vi "main2work.vi"() -> ()   [LabVIEW 2014]
uses:
  type definitions/control camera properties.ctl
  type definitions/state machine enum.ctl
  <vilib>/userdefined/High Color/IMAQdx.ctl
  <vilib>/vision/driver/NI_Vision_Acquisition_Software.lvlib
panel:
  in  "Control Camera Properties":T1={"Packet Size"=1500, "Pixel Format"=17825797, "Gain in dB"=1.0, "Exposure Time in µs"=1500, "Stream MBytes per Second"=124} {"Stream MBytes per Second" min=1 max=124 step=1 format="%#.6p"; "Exposure Time in µs" min=21 max=153391689 format="%#.0f"; "Gain in dB" min=0.0 max=26.0 format="%#_2g"; "Pixel Format" items=["Mono 12 Packed"=17563654, "Mono 12"=17825797, "Mono 8"=17301505]}
  in  "Stop Grab 2":bool
  out "Image":T2(plugin-control)
  in  "Calibration Button":bool
  out "Image Pixels (I16)":i16[][](array[numeric])
  out "Camera":T3
  in  "select camera":bool
  in  "Stop Button":bool
  in  "Snap Button":bool
  in  "Grab Button":bool
  in  "Save As Button":bool
  in  "Save Button":bool
  # "Bytes"
  # "Trigger"
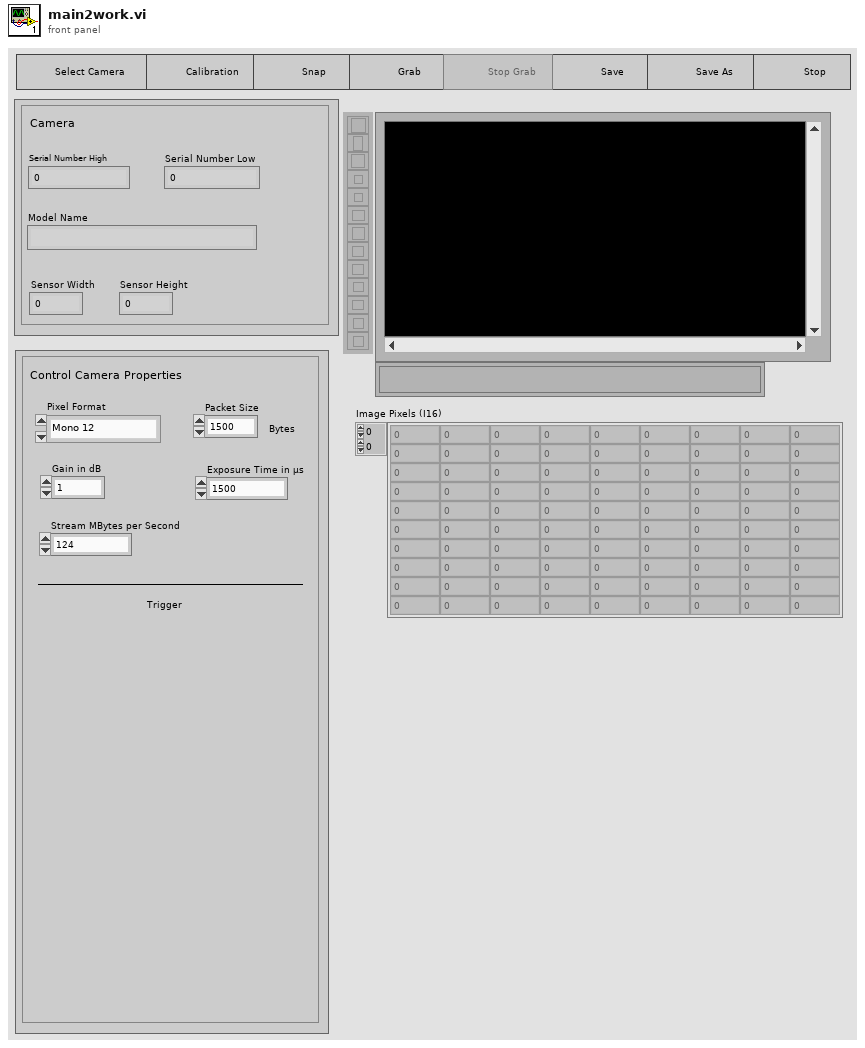
[diagram p1: front panel]
types:
  T1 = typedef "control camera properties.ctl" = cluster{"Packet Size":u32, "Pixel Format":u32, "Gain in dB":dbl, "Exposure Time in µs":u32, "Stream MBytes per Second":u32}
  T2 = typedef "IMAQ Image.ctl" = refnum<image>
  T3 = cluster{"Serial Number High":u32, "Model Name":string, "Sensor Width":u32, "Sensor Height":u32, "Serial Number Low":u32}
  T4 = cluster{"Packet Size":u32, "Pixel Format":u32, "Gain in dB":dbl, "Exposure Time in µs":u32, "Stream Bytes per Second":u32}
  T5 = typedef "IMAQdx.ctl" = refnum<k21>
  T6 = typedef "state machine enum.ctl" = enum16{"start", "select camera", "control camera properties", "calibration", "wait", "snap", "save", "save as", "grab", "error", "stop"}
  T7 = enum8{"Enabled", "Disabled", "Disabled and Grayed Out"}
  T8 = cluster{"Serial Number High":bool, "Model Name":bool, "Sensor Width":bool, "Sensor Height":bool, "Serial Number Low":bool}
  T9 = typedef "Image Type" = u32
  T10 = cluster{"PixelFormat":u32, "PacketSize":u32, "ValueDBL":dbl, "ValueU32":u32, "ValueU32":u32}
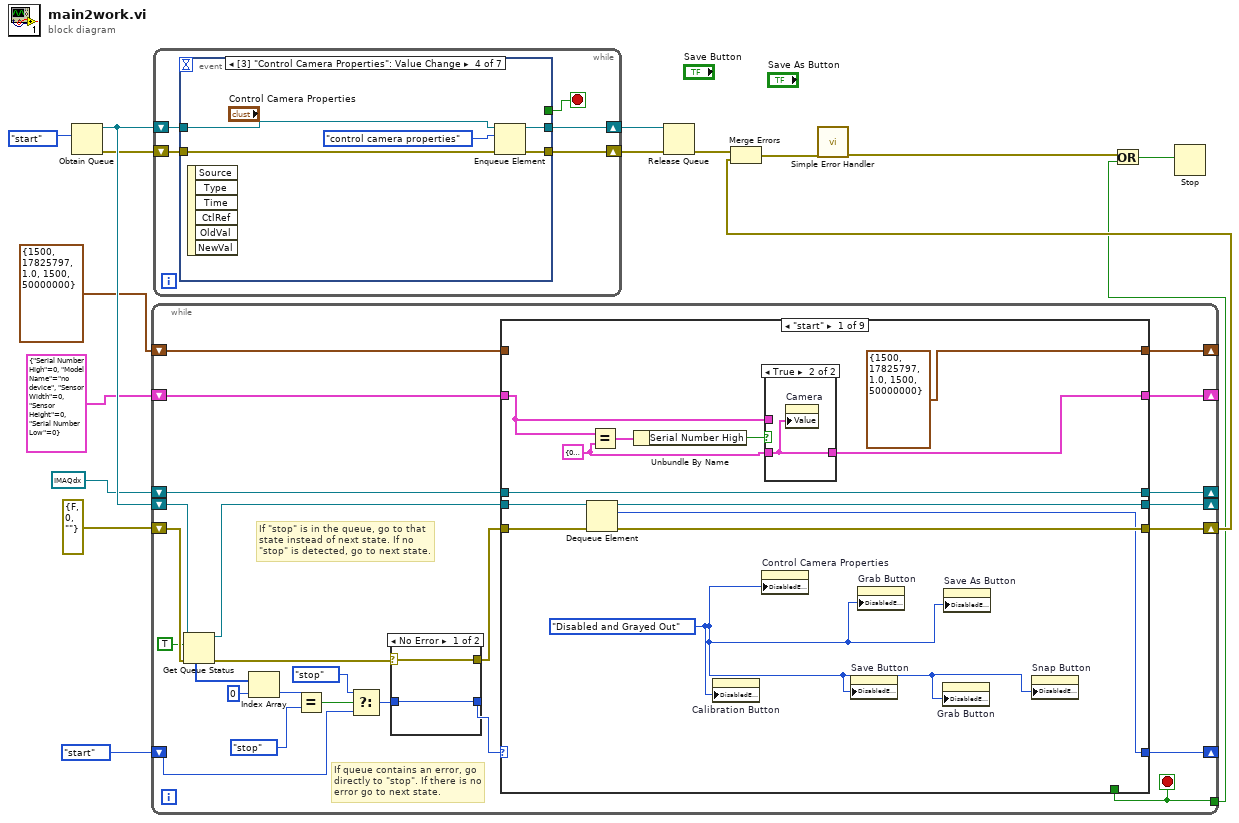
[diagram p0: block diagram]
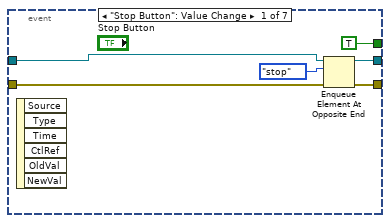
[diagram p2: hidden frame]
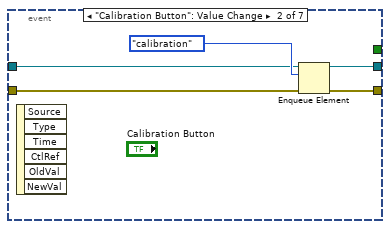
[diagram p3: hidden frame]
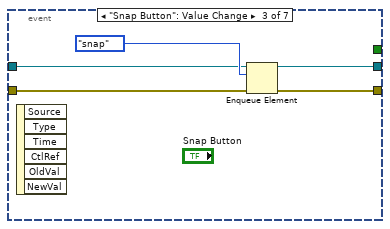
[diagram p4: hidden frame]
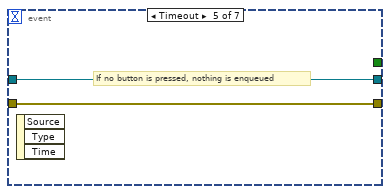
[diagram p5: hidden frame]
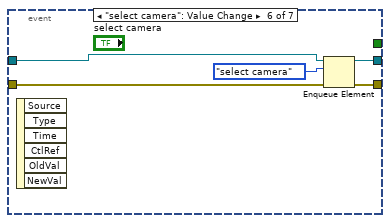
[diagram p6: hidden frame]
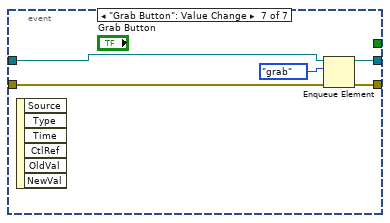
[diagram p7: hidden frame]
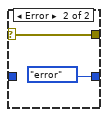
[diagram p8: hidden frame]
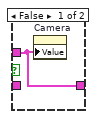
[diagram p9: hidden frame]
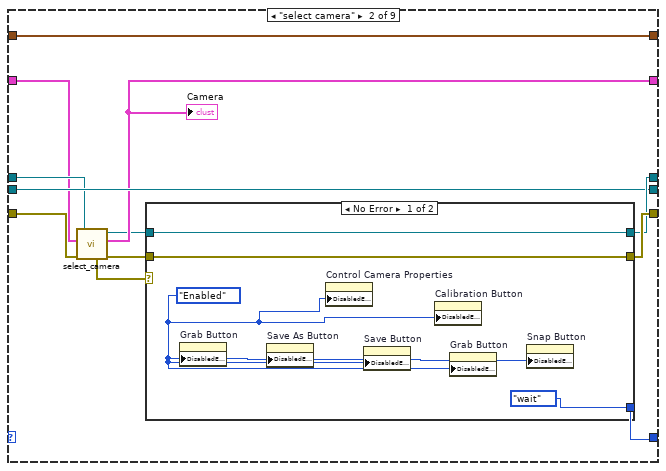
[diagram p10: hidden frame]
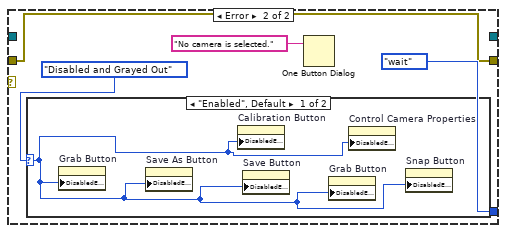
[diagram p11: hidden frame]
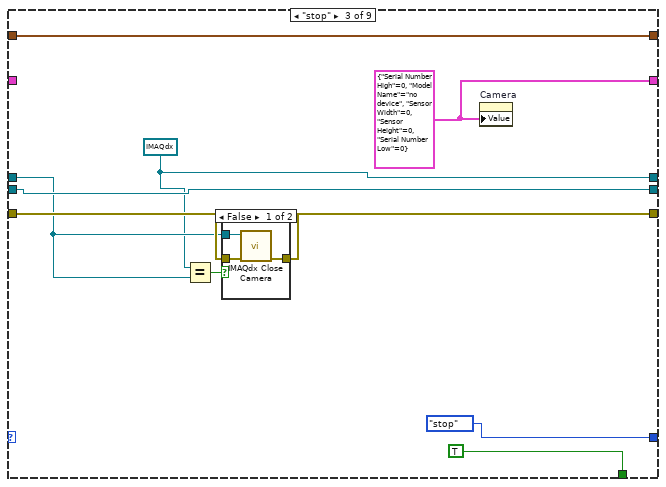
[diagram p13: hidden frame]
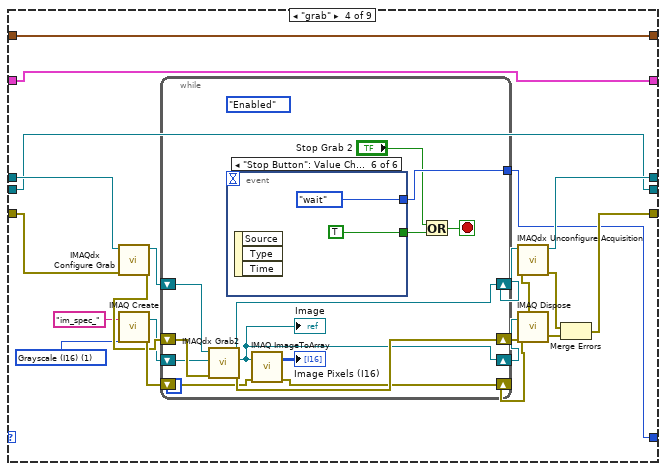
[diagram p15: hidden frame]
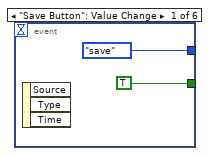
[diagram p16: hidden frame]
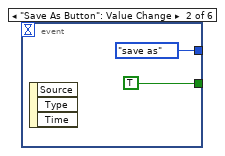
[diagram p17: hidden frame]
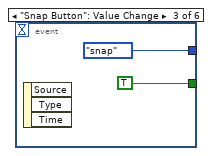
[diagram p18: hidden frame]
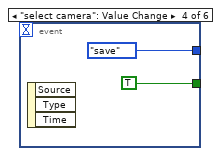
[diagram p19: hidden frame]
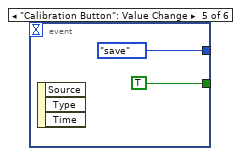
[diagram p20: hidden frame]
diagram:
  n1 = Obtain Queue(element data type=state_machine_enum."start" ("Zustände")) -> (queue out=w15:refnum<queue>, error out=w5:errorcluster)  [unwired: 4 in, 1 out]
  n2 = while {
    shift-right: [w17] -> _
    shift-left: T4 {"Packet Size"=1500, "Pixel Format"=17825797, "Gain in dB"=1.0, "Exposure Time in µs"=1500, "Stream Bytes per Second"=50000000} ("Control Camera Properties 3") -> [w41]
    shift-right: [w37] -> w11
    shift-left: errorcluster {"status"=FALSE, "code"=0, "source"=""} ("error out") -> [w32]
    shift-right: [w40] -> _
    shift-left: state_machine_enum."start" ("Zustände") -> [w25]
    shift-right: [w39] -> _
    shift-left: T5 refnum ("Session Out 2") -> [w38]
    shift-right: [w36] -> _
    shift-left: w15 -> [w34]
    tunnel: [w35] -> w4
    shift-right: [w19] -> _
    shift-left: T3 {"Serial Number High"=0, "Model Name"="no device", "Sensor Width"=0, "Sensor Height"=0, "Serial Number Low"=0} ("Camera 2") -> [w18]
    stop <- w35 stop-if-true
    # "If queue contains an error, go\ndirectly to \"stop\". If there is no\nerror go to next state."
    # "If \"stop\" is in the queue, go to that \nstate instead of next state. If no\n\"stop\" is detected, go to next state."
    n3 = Get Queue Status(queue=w34, return elements? (F)=TRUE, error in (no error)=w32) -> (queue out=w33:refnum<queue>, error out=w23:errorcluster, elements=w28:T6[])  [unwired: 5 out]
    n4 = Index Array(array=w28, index=0) -> (element=w30:T6)
    n5 = Equal?(x=w30, y=state_machine_enum."stop" ("Zustände")) -> (x = y?=w31:bool)
    n6 = Select(t=state_machine_enum."stop" ("Zustände"), s=w31, f=w25) -> (s? t:f=w20:T6)
    n7 = case shown="No Error" w23 {
      selector: w23 -> [w43 w44]
      tunnel: [w43 w44] -> w22
      tunnel: [w42 state_machine_enum."error" ("Zustände")] -> w21
      tunnel: w20 -> [w42 _]
      frame No Error {
      }
      frame Error {
      }
    }
    n8 = case shown="\"start\"" w21 {
      selector: w21 -> [_ _ _ _ _ w162 _ _ _]
      tunnel: [T4 {"Packet Size"=1500, "Pixel Format"=17825797, "Gain in dB"=1.0, "Exposure Time in µs"=1500, "Stream Bytes per Second"=50000000} ("Control Camera Properties 3") w72 w84 w98 w143 w154 _ w176 w183] -> w17
      tunnel: w41 -> [_ w72 w84 w98 w143 _ _ w176 w183]
      tunnel: w22 -> [w57 w64 w90 w102 w148 w165 w171 w172 w190]
      tunnel: [w48 w70 state_machine_enum."stop" ("Zustände") w96 w145 w157 state_machine_enum."error" ("Zustände") state_machine_enum."wait" ("Zustände") state_machine_enum."wait" ("Zustände")] -> w40
      tunnel: [_ _ TRUE _ _ _ _ _ _] -> w35
      tunnel: [w58 w69 w82 w101 w142 w164 _ w174 w186] -> w39
      tunnel: w38 -> [w58 w67 w88 w103 w142 w166 w170 w174 w191]
      tunnel: [w55 w71 w86 w100 w146 w163 _ w172 w184] -> w37
      tunnel: [w54 w68 w91 w99 w147 w156 _ w173 w181] -> w36
      tunnel: w33 -> [w56 w68 w91 w99 w149 w156 _ w173 w181]
      tunnel: [w49 w63 w83 w97 w141 w155 _ w175 w182] -> w19
      tunnel: w18 -> [w50 w62 _ w97 w141 w155 _ w175 w182]
      frame "start" {
        w51 = T3 {"Serial Number High"=0, "Model Name"="no device", "Sensor Width"=0, "Sensor Height"=0, "Serial Number Low"=0} ("Camera 2")
        w46 = T7."Disabled and Grayed Out" ("Disabled")
        n9 = Dequeue Element(queue=w56, error in (no error)=w57) -> (queue out=w54:refnum<queue>, element=w48:T6, error out=w55:errorcluster)  [unwired: 1 in, 1 out]
        n10 = Equal?(x=w50, y=w51) -> (x = y?=w53:T8)
        n11 = Unbundle By Name(w53) -> ("Serial Number High"=w52:bool)
        n12 = property on="Calibration Button" class="Bool"("DisabledEnum"=w46) -> ()  [unwired: 2 in, 2 out]
        n13 = property on="Control Camera Properties" class="Clust (strict)"("DisabledEnum"=w46) -> ()  [unwired: 2 in, 2 out]
        n14 = case shown="True" w52 {
          tunnel: w51 -> [_ w60]
          tunnel: w50 -> [w59 _]
          tunnel: [w59 w60] -> w49
          frame False {
            n15 = property on="Camera" class="Clust (strict)"("Value"=w59) -> ()  [unwired: 2 in, 2 out]
          }
          frame True {
            n16 = property on="Camera" class="Clust (strict)"("Value"=w60) -> ()  [unwired: 2 in, 2 out]
          }
        }
        n17 = property on="Save Button" class="Bool"("DisabledEnum"=w46) -> ()  [unwired: 2 in, 2 out]
        n18 = property on="Grab Button" class="Bool"("DisabledEnum"=w46) -> ()  [unwired: 2 in, 2 out]
        n19 = property on="Grab Button" class="Bool"("DisabledEnum"=w46) -> ()  [unwired: 2 in, 2 out]
        n20 = property on="Save As Button" class="Bool"("DisabledEnum"=w46) -> ()  [unwired: 2 in, 2 out]
        n21 = property on="Snap Button" class="Bool"("DisabledEnum"=w46) -> ()  [unwired: 2 in, 2 out]
      }
      frame "select camera" {
        n22 = call "select_camera.vi"("error in (no error)"=w64, "Chosen Camera: 2"=w62, "Session In"=w67) -> ("error out"=w66:errorcluster, "Chosen Camera:"=w63:T3, "Session Out"=w61:T5, "Session error"=w65:errorcluster)  [unwired: 5 in]
        "Camera" <- w63
        n23 = case shown="No Error" w65 {
          tunnel: w61 -> [w75 _]
          tunnel: w66 -> [w76 w77]
          tunnel: [w75 _] -> w69
          tunnel: [w76 w77] -> w71
          tunnel: [state_machine_enum."wait" ("Zustände") state_machine_enum."wait" ("Zustände")] -> w70
          frame No Error {
            w73 = T7."Enabled" ("Disabled")
            n24 = property on="Grab Button" class="Bool"("DisabledEnum"=w73) -> ()  [unwired: 2 in, 2 out]
            n25 = property on="Save As Button" class="Bool"("DisabledEnum"=w73) -> ()  [unwired: 2 in, 2 out]
            n26 = property on="Control Camera Properties" class="Clust (strict)"("DisabledEnum"=w73) -> ()  [unwired: 2 in, 2 out]
            n27 = property on="Save Button" class="Bool"("DisabledEnum"=w73) -> ()  [unwired: 2 in, 2 out]
            n28 = property on="Calibration Button" class="Bool"("DisabledEnum"=w73) -> ()  [unwired: 2 in, 2 out]
            n29 = property on="Grab Button" class="Bool"("DisabledEnum"=w73) -> ()  [unwired: 2 in, 2 out]
            n30 = property on="Snap Button" class="Bool"("DisabledEnum"=w73) -> ()  [unwired: 2 in, 2 out]
          }
          frame Error {
            n31 = case shown="\"Enabled\", Default" T7."Disabled and Grayed Out" ("Disabled") {
              selector: T7."Disabled and Grayed Out" ("Disabled") -> [w81 _]
              frame "Enabled", Default {
                n32 = property on="Grab Button" class="Bool"("DisabledEnum"=w81) -> ()  [unwired: 2 in, 2 out]
                n33 = property on="Save As Button" class="Bool"("DisabledEnum"=w81) -> ()  [unwired: 2 in, 2 out]
                n34 = property on="Calibration Button" class="Bool"("DisabledEnum"=w81) -> ()  [unwired: 2 in, 2 out]
                n35 = property on="Save Button" class="Bool"("DisabledEnum"=w81) -> ()  [unwired: 2 in, 2 out]
                n36 = property on="Grab Button" class="Bool"("DisabledEnum"=w81) -> ()  [unwired: 2 in, 2 out]
                n37 = property on="Control Camera Properties" class="Clust (strict)"("DisabledEnum"=w81) -> ()  [unwired: 2 in, 2 out]
                n38 = property on="Snap Button" class="Bool"("DisabledEnum"=w81) -> ()  [unwired: 2 in, 2 out]
              }
              frame "Disabled" {
              }
            }
            n39 = One Button Dialog(message="No camera is selected.") -> ()  [unwired: 1 in, 1 out]
          }
        }
      }
      frame "stop" {
        w83 = T3 {"Serial Number High"=0, "Model Name"="no device", "Sensor Width"=0, "Sensor Height"=0, "Serial Number Low"=0} ("Camera 2")
        w82 = T5 refnum ("Session Out 2")
        n40 = Equal?(x=w82, y=w88) -> (x = y?=w89:bool)
        n41 = case shown="False" w89 {
          tunnel: w90 -> [w93 w95]
          tunnel: w88 -> [w94 _]
          tunnel: [w92 w95] -> w86
          frame False {
            n42 = call <vilib>:"IMAQdx Close Camera.vi"("error in"=w93, "Session In"=w94) -> ("error out"=w92:errorcluster)  [unwired: 9 in]
          }
          frame True {
          }
        }
        n43 = property on="Camera" class="Clust (strict)"("Value"=w83) -> ()  [unwired: 2 in, 2 out]
      }
      frame "grab" {
        w105 = T9 1 items=["Grayscale (U8)", "Grayscale (I16)", "Grayscale (SGL)", "Complex (CSG)", "RGB (U32)", "HSL (U32)", "RGB (U64)", "Grayscale (U16)"] ("Image Type")
        n44 = call <vilib>:"IMAQdx Configure Grab.vi"("error in"=w102, "Session In"=w103) -> ("error out"=w108:errorcluster, "Session Out"=w104:T5)  [unwired: 8 in]
        n45 = call "IMAQ Create"("Image Name"="im_spec_", "Image Type"=w105) -> ("New Image"=w107:T2, "error out"=w112:errorcluster)  [unwired: 3 in]
        n46 = while {
          shift-right: [w120] -> w109
          shift-left: w107 -> [w124]
          shift-right: [w127] -> w110
          shift-left: w104 -> [w128]
          shift-right: [w121] -> w113
          shift-left: w112 -> [w122]
          shift-right: [w125] -> w111
          shift-left: w108 -> [w126]
          tunnel: [w119] -> w96
          stop <- w116 stop-if-true
          (unwired) T7."Enabled" ("Disabled")
          n47 = call <vilib>:"IMAQdx Grab2.vi"("error in"=w126, "Image In"=w124, "Session In"=w128) -> ("error out"=w125:errorcluster, "Image Out"=w120:T2, "Session Out"=w127:T5)  [unwired: 5 in, 1 out]
          "Image" <- w120
          n48 = event shown="[5] \"Stop Button\": Value Change" {
            selector: _ -> [_ _ _ _ _ _]
            dyn-events: _ -> [_ _ _ _ _ _]
            timeout: _ -> [_ _ _ _ _ _]
            tunnel: [TRUE TRUE TRUE TRUE TRUE TRUE] -> w118
            tunnel: [state_machine_enum."save" ("Zustände") state_machine_enum."save as" ("Zustände") state_machine_enum."snap" ("Zustände") state_machine_enum."save" ("Zustände") state_machine_enum."save" ("Zustände") state_machine_enum."wait" ("Zustände")] -> w119
            event "Save Button": Value Change {
              n49 = event-data() -> ()  [unwired: 1 in, 3 out]
            }
            event "Save As Button": Value Change {
              n50 = event-data() -> ()  [unwired: 1 in, 3 out]
            }
            event "Snap Button": Value Change {
              n51 = event-data() -> ()  [unwired: 1 in, 3 out]
            }
            event "select camera": Value Change {
              n52 = event-data() -> ()  [unwired: 1 in, 3 out]
            }
            event "Calibration Button": Value Change {
              n53 = event-data() -> ()  [unwired: 1 in, 3 out]
            }
            event "Stop Button": Value Change {
              n54 = event-data() -> ()  [unwired: 1 in, 3 out]
            }
          }
          n55 = call "IMAQ ImageToArray"("error in (no error)"=w122, "Image"=w120) -> ("error out"=w121:errorcluster, "Image Pixels (I16)"=→"Image Pixels (I16)":i16[][])  [unwired: 2 in, 3 out]
          n56 = Or(x="Stop Grab 2", y=w118) -> (x .or. y?=w116:bool)
        }
        n57 = call <vilib>:"IMAQdx Unconfigure Acquisition.vi"("error in"=w111, "Session In"=w110) -> ("error out"=w114:errorcluster, "Session Out"=w101:T5)  [unwired: 8 in]
        n58 = call "IMAQ Dispose"("Image"=w109, "error in (no error)"=w113) -> ("error out"=w115:errorcluster)  [unwired: 4 in]
        n59 = Merge Errors(w114, w115) -> (w100:errorcluster)
      }
      frame "wait", Default {
        # "If no element in queue, go back to wait state,\nto wait for another element to enqueue. If there\nis an element in queue, go to next Process"
        # "Dequeue Next Process in queue"
        n60 = Dequeue Element(queue=w149, error in (no error)=w148) -> (queue out=w147:refnum<queue>, element=w144:T6, timed out?=w150:bool, error out=w146:errorcluster)  [unwired: 1 in]
        n61 = case shown="False" w150 {
          tunnel: [w151 state_machine_enum."wait" ("Zustände")] -> w145
          tunnel: w144 -> [w151 _]
          frame False {
          }
          frame True {
          }
        }
      }
      frame "control camera properties" {
        n62 = property on="Control Camera Properties" class="Clust (strict)"() -> ("Value"=w153:T1)  [unwired: 2 in, 2 out]
        n63 = call "Control Camera Properties.vi"("error in (no error)"=w165, "Control Camera Properties"=w153, "IMAQdx Session"=w166) -> ("error out 2"=w163:errorcluster, "output cluster"=w154:T10, "Session Out 2"=w164:T5)  [unwired: 6 in]
        n64 = Equal?(x=w162, y=state_machine_enum."grab" ("Zustände")) -> (x = y?=w160:bool)
        n65 = Select(t=state_machine_enum."grab" ("Zustände"), s=w160, f=state_machine_enum."wait" ("Zustände")) -> (s? t:f=w157:T6)
      }
      frame "error" {
        n66 = call <vilib>:"IMAQdx Close Camera.vi"("error in"=w171, "Session In"=w170) -> ("error out"=w169:errorcluster)  [unwired: 9 in]
        n67 = call <vilib>:"General Error Handler.vi"("error in (no error)"=w169) -> ("error?"=w168:bool)  [unwired: 10 in, 4 out]
        n68 = Stop(stop? (T)=w168) -> ()
      }
      frame "calibration" {
        n69 = call "calibrate.vi"() -> ()  [unwired: 12 in]
      }
      frame "snap" {
        w193 = T9 1 items=["Grayscale (U8)", "Grayscale (I16)", "Grayscale (SGL)", "Complex (CSG)", "RGB (U32)", "HSL (U32)", "RGB (U64)", "Grayscale (U16)"] ("Image Type")
        n70 = call <vilib>:"IMAQdx Configure Grab.vi"("error in"=w190, "Session In"=w191) -> ("error out"=w189:errorcluster, "Session Out"=w188:T5)  [unwired: 8 in]
        n71 = call "IMAQ Create"("Image Name"="im_spec_", "Image Type"=w193) -> ("New Image"=w187:T2, "error out"=w178:errorcluster)  [unwired: 3 in]
        n72 = call <vilib>:"IMAQdx Snap2.vi"("error in"=w189, "Image In"=w187, "Session In"=w188) -> ("error out"=w185:errorcluster, "Image Out"=w179:T2, "Session Out"=w186:T5)  [unwired: 6 in]
        n73 = property on="Image" class="ImageControl"("Value"=w179) -> ()  [unwired: 2 in, 2 out]
        n74 = Merge Errors(w185, w178) -> (w184:errorcluster)
      }
    }
  }
  n75 = while {
    shift-right: [w197] -> w14
    shift-left: w5 -> [w195]
    shift-right: [w196] -> w6
    shift-left: w15 -> [w198]
    stop <- w194 stop-if-true
    n76 = event shown="[3] \"Control Camera Properties\": Value Change" {
      selector: _ -> [_ _ _ _ _ _ _]
      dyn-events: _ -> [_ _ _ _ _ _ _]
      timeout: _ -> [_ _ _ _ _ _ _]
      tunnel: w198 -> [w204 w208 w213 w218 w221 w225 w231]
      tunnel: [w201 w206 w211 w215 w220 w224 w229] -> w197
      tunnel: [TRUE _ _ _ _ _ _] -> w194
      tunnel: [w200 w205 w212 w217 w221 w223 w230] -> w196
      tunnel: w195 -> [w199 w207 w210 w216 w220 w222 w227]
      event "Stop Button": Value Change {
        n77 = event-data() -> ()  [unwired: 1 in, 6 out]
        n78 = Enqueue Element At Opposite End(queue=w204, element=state_machine_enum."stop" ("Zustände"), error in (no error)=w199) -> (queue out=w200:refnum<queue>, error out=w201:errorcluster)  [unwired: 1 in, 1 out]
      }
      event "Calibration Button": Value Change {
        n79 = event-data() -> ()  [unwired: 1 in, 6 out]
        n80 = Enqueue Element(queue=w208, element=state_machine_enum."calibration" ("Zustände"), error in (no error)=w207) -> (queue out=w205:refnum<queue>, error out=w206:errorcluster)  [unwired: 1 in, 1 out]
      }
      event "Snap Button": Value Change {
        n81 = event-data() -> ()  [unwired: 1 in, 6 out]
        n82 = Enqueue Element(queue=w213, element=state_machine_enum."snap" ("Zustände"), error in (no error)=w210) -> (queue out=w212:refnum<queue>, error out=w211:errorcluster)  [unwired: 1 in, 1 out]
      }
      event Value Change {
        n83 = event-data() -> ()  [unwired: 1 in, 6 out]
        n84 = Enqueue Element(queue=w218, element=state_machine_enum."control camera properties" ("Zustände"), error in (no error)=w216) -> (queue out=w217:refnum<queue>, error out=w215:errorcluster)  [unwired: 1 in, 1 out]
      }
      event Timeout {
        # "If no button is pressed, nothing is enqueued"
        n85 = event-data() -> ()  [unwired: 1 in, 3 out]
      }
      event "select camera": Value Change {
        n86 = event-data() -> ()  [unwired: 1 in, 6 out]
        n87 = Enqueue Element(queue=w225, element=state_machine_enum."select camera" ("Zustände"), error in (no error)=w222) -> (queue out=w223:refnum<queue>, error out=w224:errorcluster)  [unwired: 1 in, 1 out]
      }
      event "Grab Button": Value Change {
        n88 = event-data() -> ()  [unwired: 1 in, 6 out]
        n89 = Enqueue Element(queue=w231, element=state_machine_enum."grab" ("Zustände"), error in (no error)=w227) -> (queue out=w230:refnum<queue>, error out=w229:errorcluster)  [unwired: 1 in, 1 out]
      }
    }
  }
  n90 = Release Queue(queue=w6, error in (no error)=w14) -> (error out=w10:errorcluster)  [unwired: 1 in, 2 out]
  n91 = Merge Errors(w10, w11) -> (w9:errorcluster)
  n92 = call <vilib>:"Simple Error Handler.vi"("error in (no error)"=w9) -> ("error out"=w8:errorcluster)  [unwired: 4 in, 4 out]
  n93 = Or(x=w8, y=w4) -> (x .or. y?=w12:bool)
  n94 = Stop(stop? (T)=w12) -> ()
